vi "LV Config Read.vi"   [LabVIEW 2015]
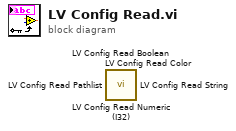
[diagram p0: block diagram]
diagram:
  n1 = call <resource>:"LV Config Read Numeric (I32).vi"() -> ()  [unwired: 5 in, 3 out]
  n2 = call <resource>:"LV Config Read Color.vi"() -> ()  [unwired: 5 in, 3 out]
  n3 = call <resource>:"LV Config Read Pathlist.vi"() -> ()  [unwired: 5 in, 3 out]
  n4 = call <resource>:"LV Config Read String.vi"() -> ()  [unwired: 5 in, 3 out]
  n5 = call <resource>:"LV Config Read Boolean.vi"() -> ()  [unwired: 5 in, 3 out]
